vi "Register Callback.vi"(8 "error in (no error)":errorcluster, 10 "Producer":refnum<class "Callback Producer.lvclass">, 11 "Callback Consumer in":refnum<class "Callback Consumer.lvclass">) -> (0 "error out":errorcluster, 3 "Callback Consumer out":refnum<class "Callback Consumer.lvclass">)   [LabVIEW 2020, in "Callback Consumer.lvclass"]
uses:
  Callback Consumer.lvclass
  Callback Producer/Callback Producer.lvclass
  Callback.vi
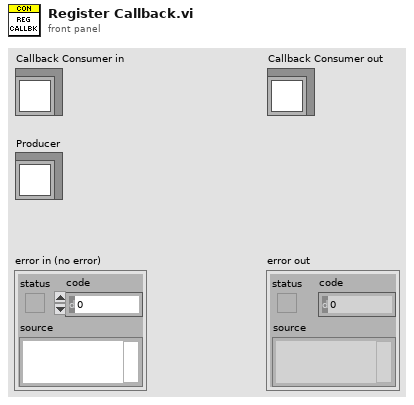
[diagram p1: front panel]
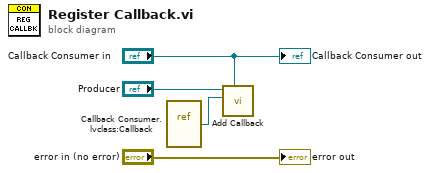
[diagram p0: block diagram]
diagram:
  n1 = vi-ref "Callback Consumer.lvclass:Callback.vi"() -> (w2:refnum<vi>)
  n2 = call "Add Callback.vi"("Owner"="Callback Consumer in", "Callback"=w2, "Callback Producer in"="Producer") -> ()  [unwired: 7 in, 2 out]
  "error out" <- "error in (no error)"
  "Callback Consumer out" <- "Callback Consumer in"
